vi "read_serie_monitor .vi"() -> ()   [LabVIEW 2016]
uses:
  <vilib>/Instr/_visa.llb/VISA Configure Serial Port (Instr).vi
panel:
  out "read buffer":string
  out "Waveform Chart":cluster{i32, i32}(graph)
  in  "baud rate":u32=9600
  in  "COM Port":refnum<visa-resource-name>
  in  "stop":bool
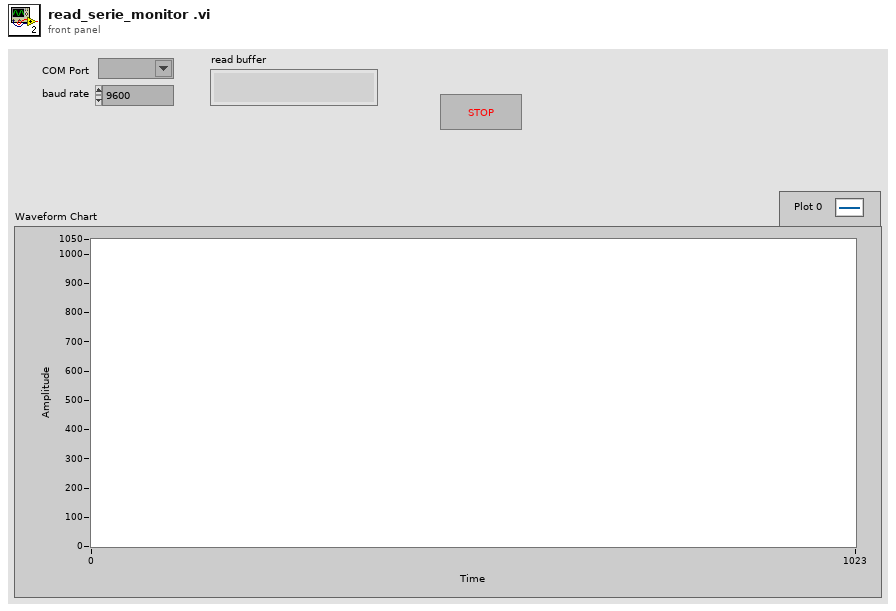
[diagram p1: front panel]
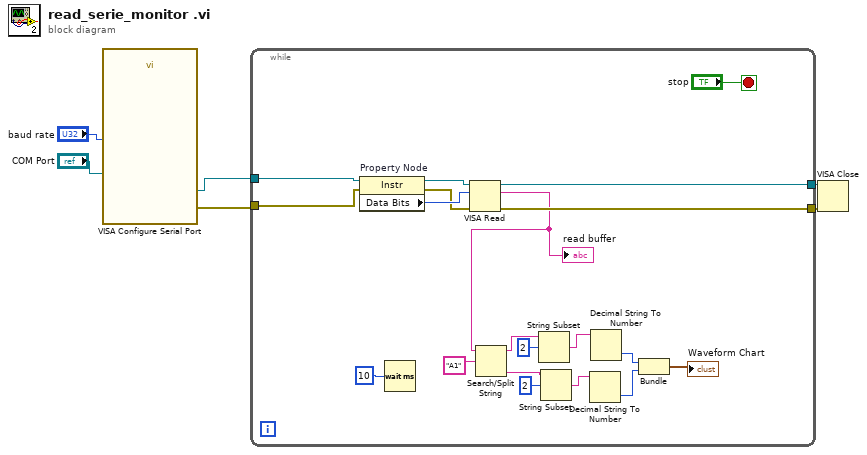
[diagram p0: block diagram]
diagram:
  n1 = call-poly "VISA Configure Serial Port"("VISA resource name"="COM Port", "baud rate (9600)"="baud rate") -> ("VISA resource name out"=w5:refnum<visa-resource-name>, "error out"=w4:errorcluster)  [unwired: 12 in]
  n2 = while {
    tunnel: w5 -> [w21]
    tunnel: w4 -> [w20]
    tunnel: [w19] -> w2
    tunnel: [w18] -> w1
    stop <- "stop" stop-if-true
    n3 = property on="Property Node" class="Instr"(reference=w21, error in=w20) -> (reference out=w23:refnum<visa-resource-name>, error out=w24:errorcluster, "Data Bits"=w25:u16)
    n4 = Wait (ms)(milliseconds to wait=u32 10) -> ()  [unwired: 1 out]
    n5 = VISA Read(VISA resource name=w23, byte count=w25, error in (no error)=w24) -> (VISA resource name out=w19:refnum<visa-resource-name>, read buffer=w12:string, error out=w18:errorcluster)  [unwired: 1 out]
    "read buffer" <- w12
    n6 = Search/Split String(string=w12, search string/char (-)="A1") -> (substring before match=w16:string, match + rest of string=w13:string)  [unwired: 1 in, 1 out]
    n7 = String Subset(string=w16, offset (0)=2) -> (substring=w11:string)  [unwired: 1 in]
    n8 = String Subset(string=w13, offset (0)=2) -> (substring=w10:string)  [unwired: 1 in]
    n9 = Decimal String To Number(string=w10) -> (number=w7:i32)  [unwired: 2 in, 1 out]
    n10 = Decimal String To Number(string=w11) -> (number=w8:i32)  [unwired: 2 in, 1 out]
    n11 = Bundle(w8, w7) -> (→"Waveform Chart":cluster{i32, i32})  [unwired: 1 in]
  }
  n12 = VISA Close(VISA resource name=w2, error in (no error)=w1) -> ()  [unwired: 1 out]
